vi "Set Interface Configuration.vi"(8 "error in (no error)":errorcluster, 9 "Value (0)":string="0", 10 "Configuration Parameter (RS-232 Enable/Disable)":i32(ring) items=["RS-232 Enable/Disable", "RS-232 Baud Rate", "GPIB Enable/Disable", "GPIB Address", "LAN TCP/IP Enable/Disable", "DHCP Enable/Disable", "Auto-Ip Enable/Disable", "Static Ip Enable/Disable", "Bare Socket Enable/Disable", "Telnet Enable/Disable", "VXI-11 Net Instrument Enable/Disable", "Static IP Address", "Subnet Address/Network Mask", "Default Gateway"], 11 "VISA resource name":refnum<visa-resource-name>) -> (0 "error out":errorcluster, 3 "VISA resource name out":refnum<visa-resource-name>, 4 "Device Errors":cluster{"code":i32, "Text":string}[](array[cluster]))   [LabVIEW 2014, in "Stanford Research DG645 - Driver.lvlib"]
doc: "Interface Command: IFCF i,j\nInstrument Error Check\n\nSet the interface configuration parameter i to j. The parameter i may be one of the following:\n\ni Configuration Parameter\n0 RS-232 Enable/Disable\n1 RS-232 Baud rate\n2 GPIB Enable/Disable\n3 GPIB Address\n4 LAN TCP/IP Enable/Disable\n5 DHCP Enable/Disable\n6 Auto-Ip Enable/Disable\n7 Static Ip Enable/Disable\n8 Bare Socket Enable/Disable\n9 Telnet Enable/Disable\n10 VXI-11 Net Instrument Enable/Disable\n11 Static IP Address\n12 Subnet Address/Network Mask\n13 Default Gateway\n\nSet j to 0 to disable and 1 to enable it. \n\nValid RS-232 baud rates include 4800, 9600, 19200, 38400, 57600, and 115200. \n\nValid GPIB addresses are in the range 0-30. \n\nParameters 10-12 require an IP address in the form a.b.c.d where each letter is a decimal integer in the range 0-255."
uses:
  Stanford Research DG645 - Driver.lvlib
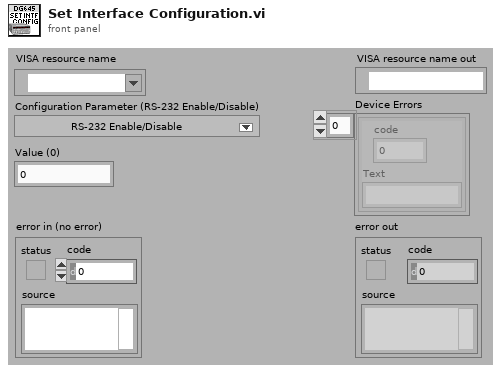
[diagram p1: front panel]
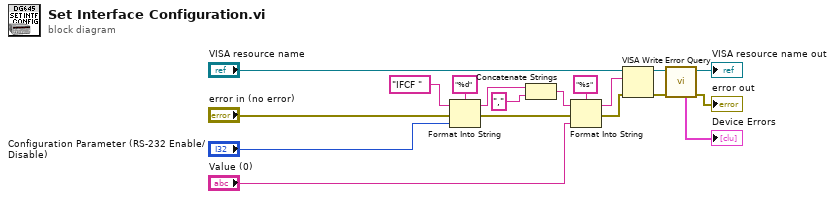
[diagram p0: block diagram]
diagram:
  n1 = Format Into String(format string="%d", initial string="IFCF " ("command"), error in="error in (no error)", "Configuration Parameter (RS-232 Enable/Disable)") -> (resulting string=w13:string, error out=w14:errorcluster)
  n2 = Concatenate Strings(w13, "," ("command")) -> (w9:string)
  n3 = Format Into String(format string="%s", initial string=w9, error in=w14, "Value (0)") -> (resulting string=w3:string, error out=w4:errorcluster)
  n4 = VISA Write(VISA resource name="VISA resource name", write buffer=w3, error in (no error)=w4) -> (VISA resource name out=w7:refnum<visa-resource-name>, error out=w6:errorcluster)  [unwired: 1 out]
  n5 = call "Error Query.vi"("error in (no error)"=w6, "VISA resource name"=w7) -> ("error out"=→"error out":errorcluster, "VISA resource name out"=→"VISA resource name out":refnum<visa-resource-name>, "Device Errors"=→"Device Errors":cluster{"code":i32, "Text":string}[])  [unwired: 7 in]
